vi "z-wave-1.vi"(2 "index":i32, 3 "amplitutude":dbl) -> (0 "Waveform Graph":dbl[](graph), 1 "array size":i32)   [LabVIEW 2012]
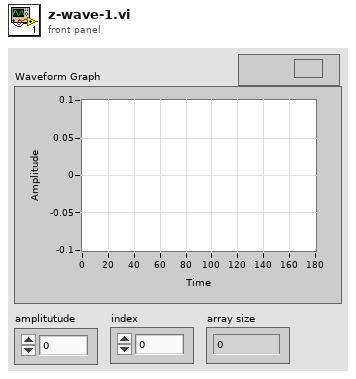
[diagram p1: front panel]
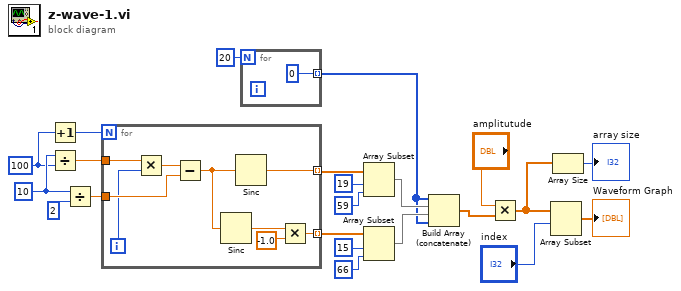
[diagram p0: block diagram]
diagram:
  w8 = 100 ("density")
  w21 = 10
  n1 = Increment(x=w8) -> (x+1=w18:i32)
  n2 = Divide(x=w21, y=w8) -> (x/y=w20:dbl)
  n3 = Divide(x=w21, y=2) -> (x/y=w19:dbl)
  n4 = for {
    N: w18 -> [_]
    tunnel: w20 -> [w31]
    tunnel: w19 -> [w30]
    tunnel: [w24] -> w17 mode=indexing
    tunnel: [w23] -> w16 mode=indexing
    i -> [w28]
    n5 = Multiply(x=w31, y=w28) -> (x*y=w29:dbl)
    n6 = Subtract(x=w29, y=w30) -> (x-y=w27:dbl)
    n7 = Sinc(1:w27) -> (0:w26:dbl)
    n8 = Sinc(1:w27) -> (0:w24:dbl)
    n9 = Multiply(x=w26, y=-1.0) -> (x*y=w23:dbl)
  }
  n10 = for {
    N: 20 -> [_]
    tunnel: [0] -> w5 mode=indexing
  }
  n11 = Array Subset(array=w17, index=19 ("index 2"), length=59) -> (w14:dbl[])
  n12 = Array Subset(array=w16, index=15 ("index 2"), length=66 ("length 2")) -> (w11:dbl[])
  n13 = Build Array (concatenate)(w5, w14, w11, w5) -> (w15:dbl[])
  n14 = Multiply(x="amplitutude", y=w15) -> (x*y=w2:dbl[])
  n15 = Array Subset(array=w2, index="index") -> (→"Waveform Graph":dbl[])  [unwired: 1 in]
  n16 = Array Size(array=w2) -> (size(s)=→"array size":i32)
